vi "Terminal-Main-GearSystem.vi"(4 "ErrorQRef":refnum<queue>, 5 "ModbusNResRef":refnum<notifier>, 6 "ModbusMsgQRef":refnum<queue>, 7 "ModbusNReqRef":refnum<notifier>, 8 "error in (no error)":errorcluster caption="错误输入（无错误）", 11 "GearSystemNRef":refnum<notifier>) -> (0 "error out":errorcluster caption="错误输出")   [LabVIEW 2014]
panel:
  out "Gear System is running":bool
  out "GearSys开始通知器":refnum<notifier>
  out "GearSys开始响应器":refnum<notifier>
  out "GearSys停止通知器":refnum<notifier>
  out "GearSys停止响应器":refnum<notifier>
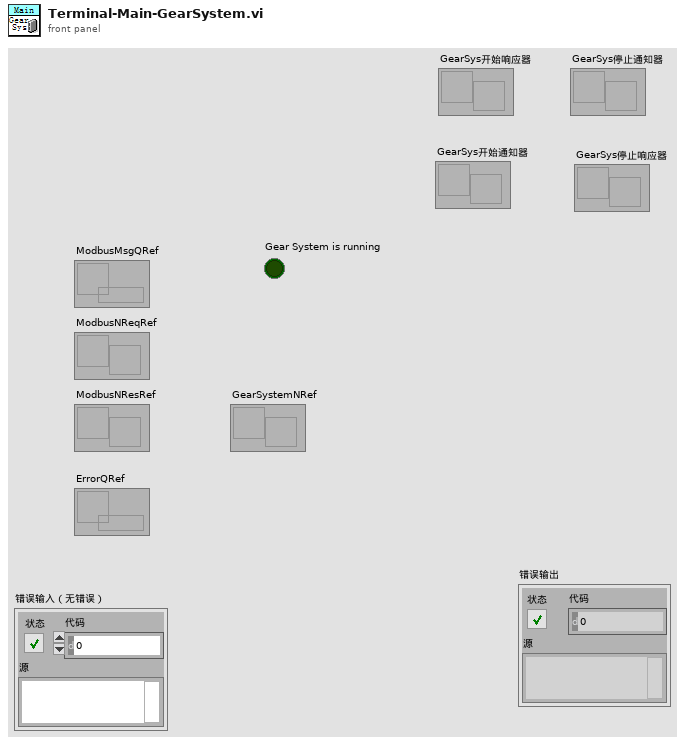
[diagram p1: front panel]
types:
  T1 = cluster{"Transaction ID":u16, "Unit ID":u8, "Starting Address":u16, "Quantity":u16}
  T2 = cluster{"Transaction ID":u16, "Unit ID":u8, "Address":u16, "Register":u16}
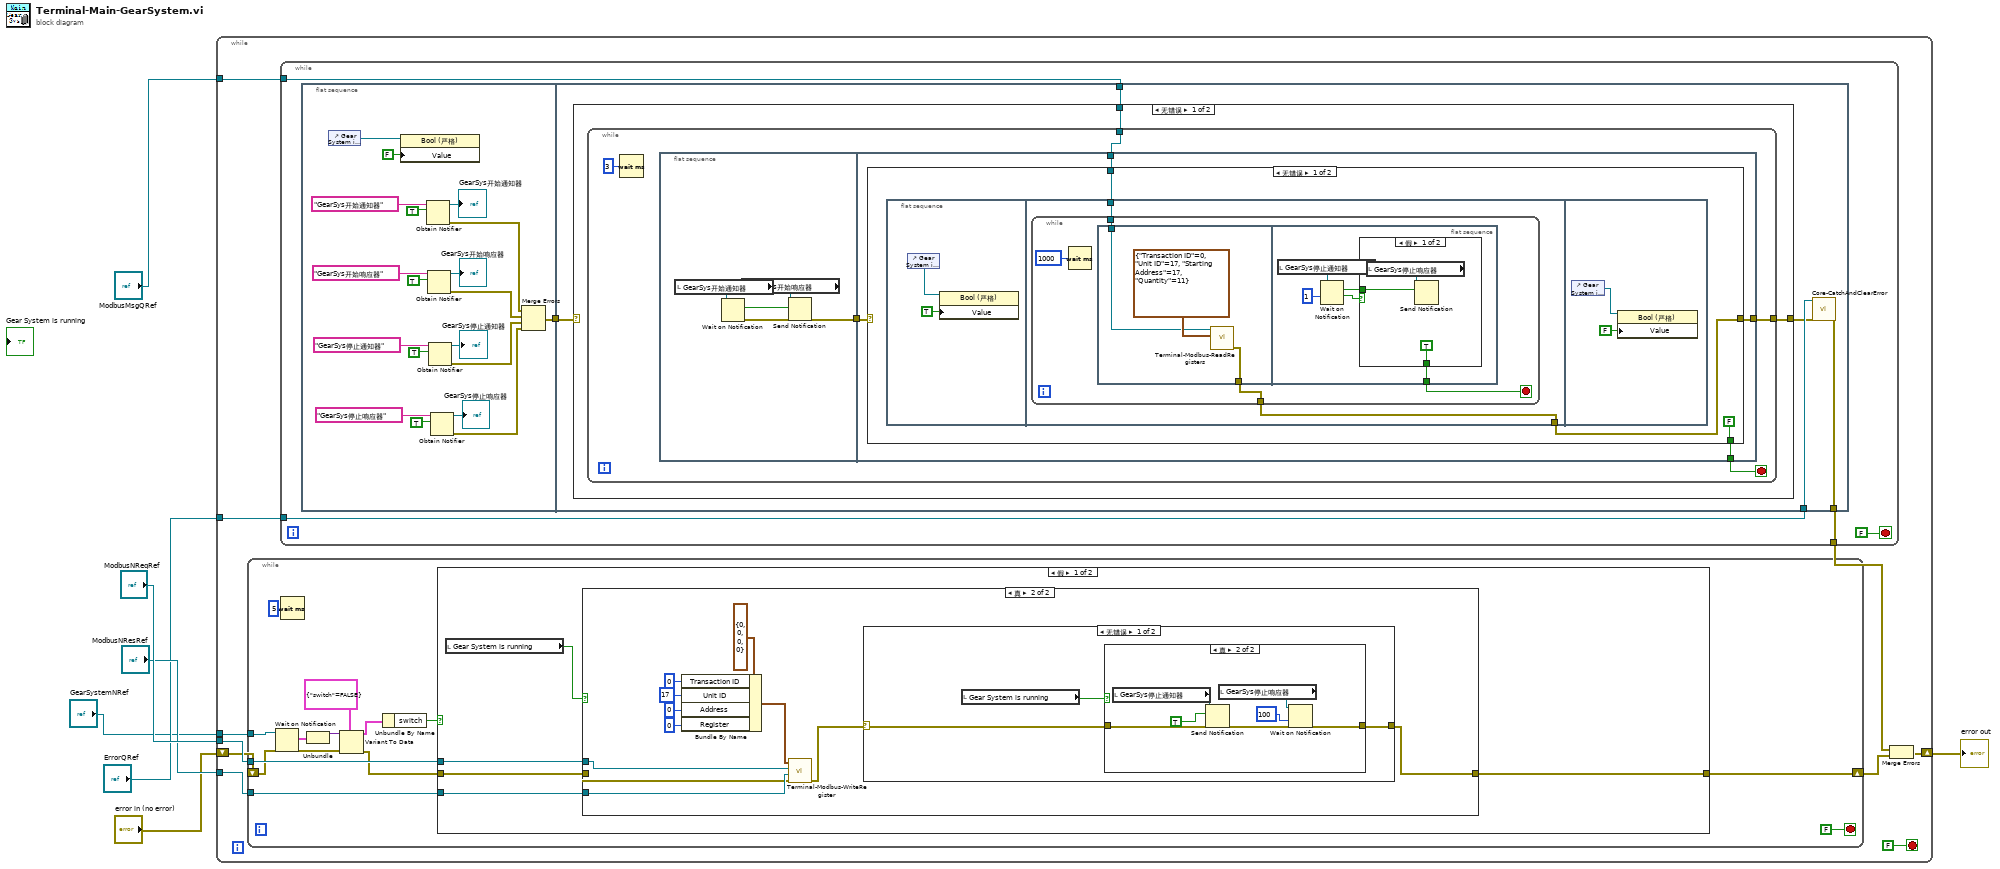
[diagram p0: block diagram]
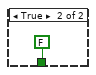
[diagram p2: hidden frame]
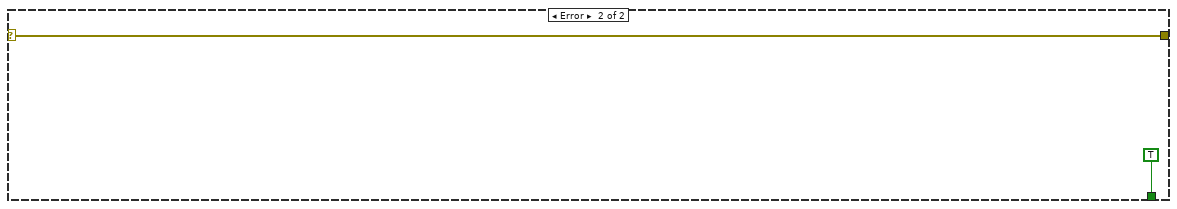
[diagram p3: hidden frame]
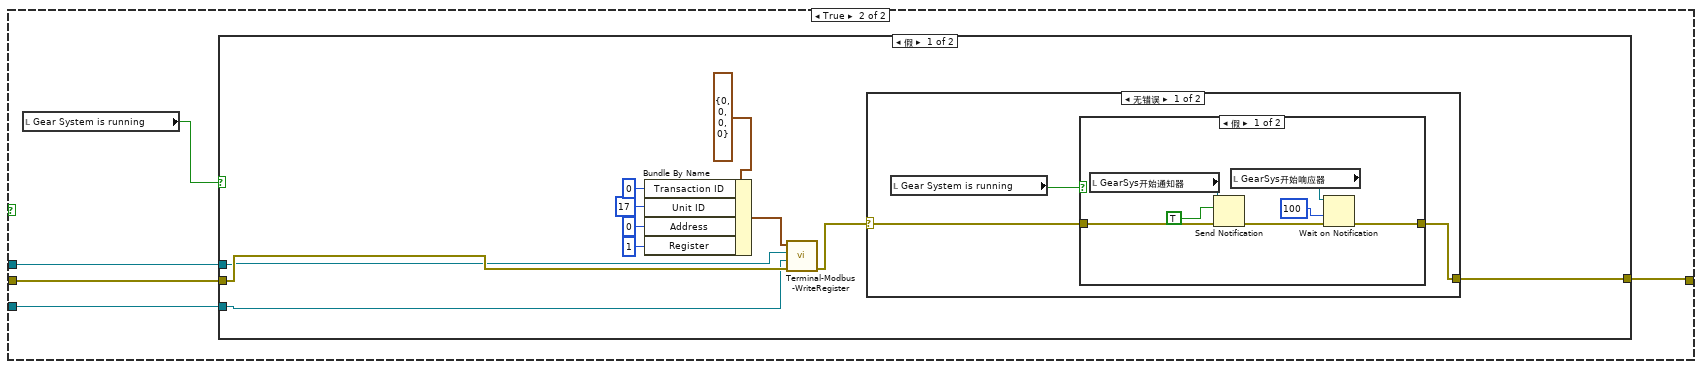
[diagram p8: hidden frame]
diagram:
  n1 = while {
    tunnel: "ModbusMsgQRef" -> [w17]
    tunnel: "ModbusNReqRef" -> [w16]
    tunnel: "ModbusNResRef" -> [w15]
    tunnel: "ErrorQRef" -> [w13]
    shift-right: [w12] -> w2
    shift-left: "error in (no error)" -> [w14]
    tunnel: "GearSystemNRef" -> [w8]
    stop <- FALSE stop-if-true
    n2 = while {
      tunnel: w16 -> [w104]
      tunnel: w15 -> [w103]
      shift-right: [w102] -> w11
      shift-left: w14 -> [w98]
      tunnel: w8 -> [w99]
      stop <- FALSE stop-if-true
      n3 = Wait on Notification(notifier=w99, error in (no error)=w98) -> (notification=w97:cluster{variant, string}, error out=w93:errorcluster)  [unwired: 2 in, 2 out]
      n4 = Wait (ms)(milliseconds to wait=u32 5 ("等待时间（毫秒）")) -> ()  [unwired: 1 out]
      n5 = Unbundle(w97) -> (w96:variant)  [unwired: 1 out]
      n6 = Variant To Data(error in=w93, type=cluster{"switch":bool} {"switch"=FALSE}, Variant=w96) -> (data=w95:cluster{"switch":bool}, error out=w92:errorcluster)
      n7 = Unbundle By Name(w95) -> ("switch"=w94:bool)
      n8 = case shown="假" w94 {
        tunnel: w104 -> [w109 w136]
        tunnel: w103 -> [w108 w137]
        tunnel: w92 -> [w107 w138]
        tunnel: [w106 w135] -> w102
        frame False {
          n9 = local read "Gear System is running"() -> (w105:bool)
          n10 = case shown="真" w105 {
            tunnel: w109 -> [_ w120]
            tunnel: w108 -> [_ w119]
            tunnel: w107 -> [w110 w118]
            tunnel: [w110 w117] -> w106
            frame False {
            }
            frame True {
              n11 = Bundle By Name(cluster=T2 {"Transaction ID"=0, "Unit ID"=0, "Address"=0, "Register"=0} ("簇"), "Transaction ID"=u16 0, "Unit ID"=u8 17, "Address"=u16 0, "Register"=u16 0) -> (w112:T2)
              n12 = call "Terminal-Modbus-WriteRegister.vi"("error in (no error)"=w118, "ModbusNResRef"=w119, "ModbusNReqRef"=w120, "簇"=w112) -> ("error out"=w121:errorcluster)  [unwired: 7 in]
              n13 = case shown="无错误" w121 {
                selector: w121 -> [w123 w133]
                tunnel: [w122 w133] -> w117
                frame No Error {
                  n14 = local read "Gear System is running"() -> (w124:bool)
                  n15 = case shown="真" w124 {
                    tunnel: [w125 w127] -> w122
                    tunnel: w123 -> [w125 w126]
                    frame False {
                    }
                    frame True {
                      n16 = local read "GearSys停止通知器"() -> (w132:refnum<notifier>)
                      n17 = Send Notification(notification=TRUE ("通知"), notifier=w132, error in (no error)=w126) -> (error out=w130:errorcluster)  [unwired: 1 out]
                      n18 = local read "GearSys停止响应器"() -> (w129:refnum<notifier>)
                      n19 = Wait on Notification(notifier=w129, timeout in ms (-1)=100 ("超时毫秒(-1)"), error in (no error)=w130) -> (error out=w127:errorcluster)  [unwired: 1 in, 3 out]
                    }
                  }
                }
                frame Error {
                }
              }
            }
          }
        }
        frame True {
          n20 = local read "Gear System is running"() -> (w134:bool)
          n21 = case shown="假" w134 {
            tunnel: w138 -> [w147 w162]
            tunnel: w137 -> [w140 _]
            tunnel: w136 -> [w139 _]
            tunnel: [w149 w162] -> w135
            frame False {
              n22 = Bundle By Name(cluster=T2 {"Transaction ID"=0, "Unit ID"=0, "Address"=0, "Register"=0} ("簇"), "Transaction ID"=u16 0, "Unit ID"=u8 17, "Address"=u16 0, "Register"=u16 1) -> (w142:T2)
              n23 = call "Terminal-Modbus-WriteRegister.vi"("error in (no error)"=w147, "ModbusNResRef"=w140, "ModbusNReqRef"=w139, "簇"=w142) -> ("error out"=w148:errorcluster)  [unwired: 7 in]
              n24 = case shown="无错误" w148 {
                selector: w148 -> [w151 w161]
                tunnel: [w150 w161] -> w149
                frame No Error {
                  n25 = local read "Gear System is running"() -> (w152:bool)
                  n26 = case shown="假" w152 {
                    tunnel: [w154 w160] -> w150
                    tunnel: w151 -> [w153 w160]
                    frame False {
                      n27 = local read "GearSys开始通知器"() -> (w159:refnum<notifier>)
                      n28 = Send Notification(notification=TRUE ("通知"), notifier=w159, error in (no error)=w153) -> (error out=w157:errorcluster)  [unwired: 1 out]
                      n29 = local read "GearSys开始响应器"() -> (w156:refnum<notifier>)
                      n30 = Wait on Notification(notifier=w156, timeout in ms (-1)=100 ("超时毫秒(-1)"), error in (no error)=w157) -> (error out=w154:errorcluster)  [unwired: 1 in, 3 out]
                    }
                    frame True {
                    }
                  }
                }
                frame Error {
                }
              }
            }
            frame True {
            }
          }
        }
      }
    }
    n31 = while {
      tunnel: w17 -> [w21]
      tunnel: w13 -> [w20]
      tunnel: [w18] -> w10
      stop <- FALSE stop-if-true
      n32 = flat-sequence {
        tunnel: [w24] -> w22
        tunnel: w22 -> [w46]
        tunnel: w20 -> [w45]
        tunnel: [w43] -> w18
        tunnel: w21 -> [w42]
        frame #0 {
          n33 = control-ref of="Gear System is running"() -> (w23:refnum<vi>)
          n34 = property class="Bool (严格)"(reference=w23, "Value"=FALSE ("值")) -> ()  [unwired: 1 in, 2 out]
          n35 = Obtain Notifier(name (unnamed)="GearSys开始通知器" ("名称（未命名）"), notification data type=TRUE) -> (notifier out=→"GearSys开始通知器":refnum<notifier>, error out=w28:errorcluster)  [unwired: 2 in, 1 out]
          n36 = Obtain Notifier(name (unnamed)="GearSys开始响应器" ("名称（未命名）"), notification data type=TRUE) -> (notifier out=→"GearSys开始响应器":refnum<notifier>, error out=w27:errorcluster)  [unwired: 2 in, 1 out]
          n37 = Obtain Notifier(name (unnamed)="GearSys停止通知器" ("名称（未命名）"), notification data type=TRUE) -> (notifier out=→"GearSys停止通知器":refnum<notifier>, error out=w26:errorcluster)  [unwired: 2 in, 1 out]
          n38 = Obtain Notifier(name (unnamed)="GearSys停止响应器" ("名称（未命名）"), notification data type=TRUE) -> (notifier out=→"GearSys停止响应器":refnum<notifier>, error out=w25:errorcluster)  [unwired: 2 in, 1 out]
          n39 = Merge Errors(w28, w27, w26, w25) -> (w24:errorcluster)
        }
        frame #1 {
          n40 = case shown="无错误" w46 {
            selector: w46 -> [_ w90]
            tunnel: [w48 w90] -> w44
            tunnel: w42 -> [w47 _]
            frame No Error {
              n41 = while {
                tunnel: [w51] -> w48
                tunnel: w47 -> [w50]
                stop <- w52 stop-if-true
                n42 = Wait (ms)(milliseconds to wait=u32 3 ("等待时间（毫秒）")) -> ()  [unwired: 1 out]
                n43 = flat-sequence {
                  tunnel: [w54] -> w53
                  tunnel: w53 -> [w62]
                  tunnel: [w61] -> w52
                  tunnel: [w60] -> w51
                  tunnel: w50 -> [w59]
                  frame #0 {
                    n44 = local read "GearSys开始通知器"() -> (w58:refnum<notifier>)
                    n45 = Wait on Notification(notifier=w58) -> (notification=w55:bool, error out=w56:errorcluster)  [unwired: 3 in, 2 out]
                    n46 = local read "GearSys开始响应器"() -> (w57:refnum<notifier>)
                    n47 = Send Notification(notification=w55, notifier=w57, error in (no error)=w56) -> (error out=w54:errorcluster)  [unwired: 1 out]
                  }
                  frame #1 {
                    n48 = case shown="无错误" w62 {
                      selector: w62 -> [_ w88]
                      tunnel: [FALSE TRUE] -> w61
                      tunnel: [w64 w88] -> w60
                      tunnel: w59 -> [w63 _]
                      frame No Error {
                        n49 = flat-sequence {
                          tunnel: [w68] -> w64
                          tunnel: w63 -> [w69]
                          frame #0 {
                            n50 = control-ref of="Gear System is running"() -> (w66:refnum<vi>)
                            n51 = property class="Bool (严格)"(reference=w66, "Value"=TRUE ("值")) -> ()  [unwired: 1 in, 2 out]
                          }
                          frame #1 {
                            n52 = while {
                              tunnel: w69 -> [w73]
                              tunnel: [w72] -> w68
                              stop <- w71 stop-if-true
                              n53 = Wait (ms)(milliseconds to wait=u32 1000 ("等待时间（毫秒）")) -> ()  [unwired: 1 out]
                              n54 = flat-sequence {
                                tunnel: w73 -> [w75]
                                tunnel: [w74] -> w72
                                tunnel: [w77] -> w71
                                frame #0 {
                                n55 = call "Terminal-Modbus-ReadRegisters.vi"("簇"=T1 {"Transaction ID"=0, "Unit ID"=17, "Starting Address"=17, "Quantity"=11}, "ModbusMsgQRef"=w75) -> ("error out"=w74:errorcluster)  [unwired: 9 in]
                                }
                                frame #1 {
                                n56 = local read "GearSys停止通知器"() -> (w80:refnum<notifier>)
                                n57 = Wait on Notification(notifier=w80, timeout in ms (-1)=1 ("超时毫秒(-1)")) -> (notification=w78:bool, timed out?=w79:bool)  [unwired: 2 in, 2 out]
                                n58 = case shown="假" w79 {
                                tunnel: [TRUE FALSE] -> w77
                                tunnel: w78 -> [w83 _]
                                frame False {
                                n59 = local read "GearSys停止响应器"() -> (w82:refnum<notifier>)
                                n60 = Send Notification(notification=w83, notifier=w82) -> ()  [unwired: 1 in, 2 out]
                                }
                                frame True {
                                }
                                }
                                }
                              }
                            }
                          }
                          frame #2 {
                            n61 = control-ref of="Gear System is running"() -> (w86:refnum<vi>)
                            n62 = property class="Bool (严格)"(reference=w86, "Value"=FALSE ("值")) -> ()  [unwired: 1 in, 2 out]
                          }
                        }
                      }
                      frame Error {
                      }
                    }
                  }
                }
              }
            }
            frame Error {
            }
          }
          n63 = call "Core-CatchAndClearError.vi"("error in (no error)"=w44, "ErrorQ"=w45) -> ("error out"=w43:errorcluster)  [unwired: 7 in]
        }
      }
    }
    n64 = Merge Errors(w10, w11) -> (w12:errorcluster)
  }
  "error out" <- w2
